vi "SimpleDemo.vi"() -> ()   [LabVIEW 2011]
uses:
  <vilib>/Platform/TimedLoop/XDataNode/timing_clust.ctl
  <vilib>/Platform/TimedLoop/XDataNode/nitl_modes.ctl
  <vilib>/Platform/TimedLoop/XDataNode/wakeup.ctl
  C:/Users/Behavior Room/Desktop/Kinect Mouse/DepthSense/FunctionPointerProxy/FunctionPointerProxy/bin/Release/FunctionPointerProxy.dll
  FunctionPointerProxy/FunctionPointerProxy/bin/Release/FunctionPointerProxy.dll
  <vilib>/Platform/TimedLoop/XDataNode/XDataNode.xnode
  <userlib>/libOptrima-2-3/libOptrima-2-3.lvlib
  <vilib>/Platform/TimedLoop/XDataNode/XDNodeRunTimeDep.lvlib
  Program Files (x86)/SoftKinetic/OptrimaSDK/lib/libOptrima-2-3.dll
panel:
  out "Image 2":T1(plugin-control)
  out "Connect Callback?":i32
  out "Disconnect Callback?":i32
  out "API version":string
  out "NewFrame Callback?":i32
  in  "stop":bool
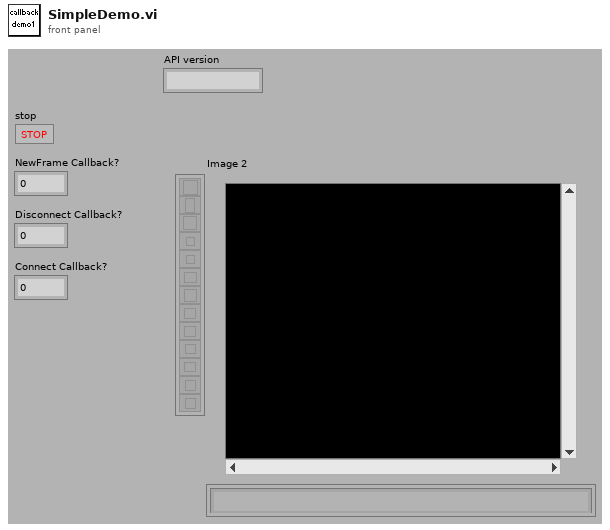
[diagram p1: front panel]
types:
  T1 = typedef "IMAQ Image.ctl" = refnum<image>
  T2 = typedef "t_CallbackReferences.ctl" = cluster{"LV event callback ":refnum<k27>, "Proxy instance":refnum<k24>, "(*f)(...)":i32}
  T3 = cluster{"queue out":refnum<queue>, "queue out":refnum<queue>}
  T4 = typedef "XDNodeRunTimeDep.lvlib/timing_clust.ctl" = cluster{"Expected End [f-1]":u64, "Actual End [f-1]":u64, "Finished Late? [f-1]":bool, "Expected End [i-1]":u64, "Actual End [i-1]":u64, "Finished Late? [i-1]":bool, "Expected Start [i]":u64, "Actual Start [i]":u64, "Expected Start [f]":u64, "Actual Start [f]":u64, "Source Name":string, "Structure Name":string, "Period":i64, "Deadline":i64, "Offset":i64, "Start":i64, "Priority":i32, "Timeout":i32, "Mode":T5, "Wakeup Reason":T6, "Error":errorcluster, "Source Type":string, "Secondary Source Type":string, "Global End Time":u64, "Global Start Time":u64, "Frame Duration":u64, "Iteration Duration":u64, "Assigned CPU":i32, "I/O Scan Engine Mode":u32}
  T5 = typedef "XDNodeRunTimeDep.lvlib/nitl_modes.ctl" = enum32{"No Change", "Process missed periods, maintain original phase", "Discard missed periods, maintain original phase", "Process missed periods, ignore original phase", "Discard missed periods, ignore original phase"}
  T6 = typedef "XDNodeRunTimeDep.lvlib/wakeup.ctl" = enum32{"Normal", "Aborted", "Asynchronous wakeup", "Timing source error", "Timed loop error", "Timeout"}
  T7 = typedef "Image Type" = u32
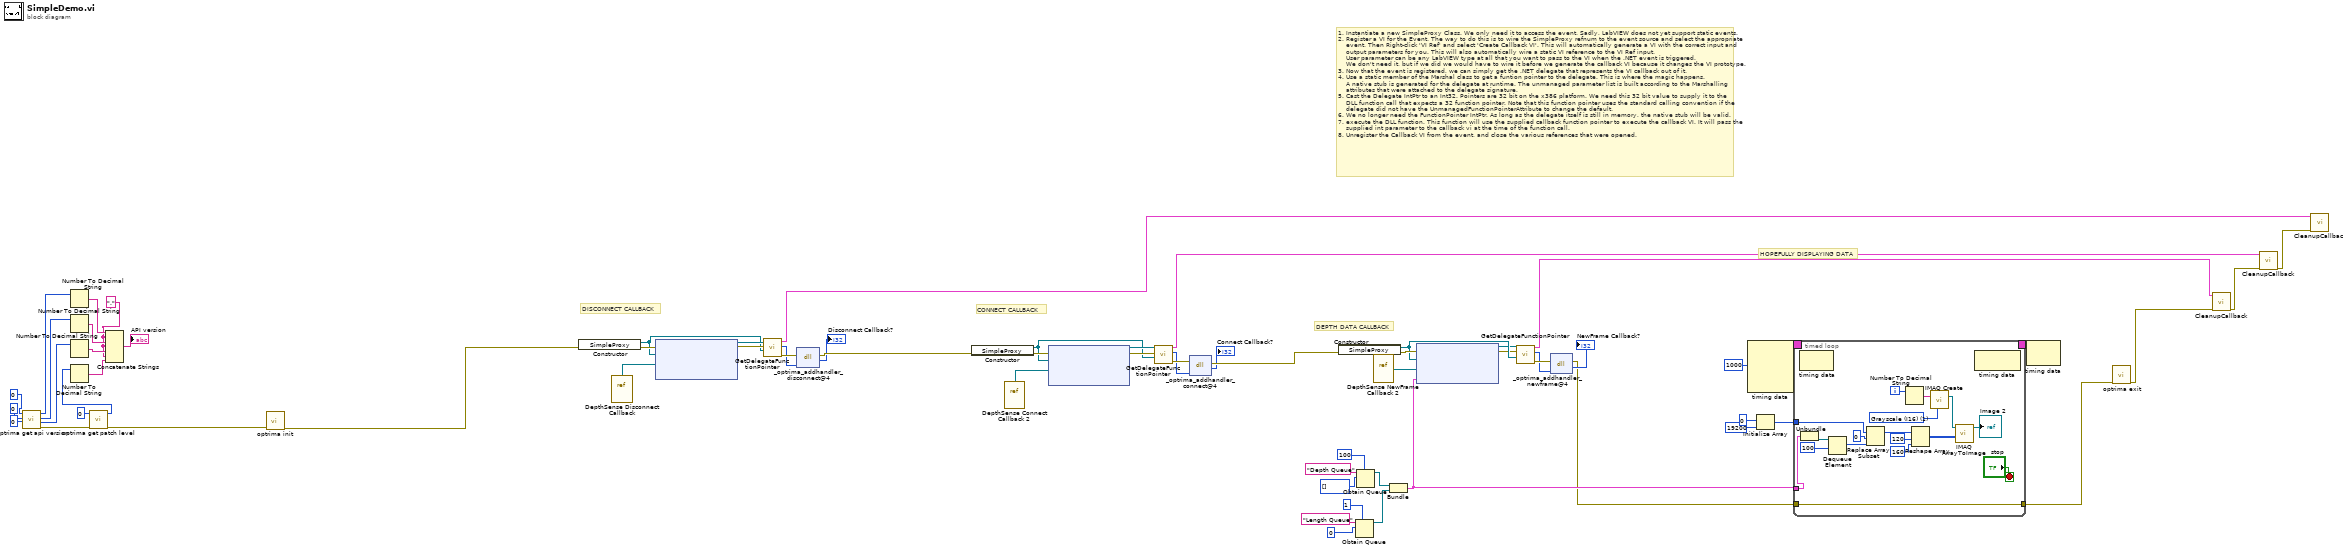
[diagram p0: block diagram]
diagram:
  w44 = "."
  # "HOPEFULLY DISPLAYING DATA"
  # "DEPTH DATA CALLBACK"
  # "CONNECT CALLBACK"
  # "DISCONNECT CALLBACK"
  # "1. Instantiate a new SimpleProxy Class. We only need it to access the event. Sadly, LabVIEW does not yet support static events.\n2. Register a VI for the Event. The way to do this is to wire the SimpleProxy refnum to the event source and select the appropriate\n    event. Then Right-click 'VI Ref' and select 'Create Callback VI'. This will automatically generate a VI with the correct input and\n    output parameters for you. This will also automatically wire a static VI reference to the VI Ref input.\n    User parameter can be any LabVIEW type at all that you want to pass to the VI when the .NET event is triggered.\n    We don't need it, but if we did we would have to wire it before we generate the callback VI because it changes the VI prototype.\n3. Now that the event is registered, we can simply get the .NET delegate that represents the VI callback out of it.\n4. Use a static member of the Marshal class to get a funtion pointer to the delegate. This is where the magic happens.\n    A native stub is generated for the delegate at runtime. The unmanaged parameter list is built according to the Marshalling\n    attributes that were attached to the delegate signature.\n5. Cast the Delegate IntPtr to an Int32. Pointers are 32 bit on the x386 platform. We need this 32 bit value to supply it to the\n    DLL function call that expects a 32 function pointer. Note that this function pointer uses the standard calling convention if the\n    delegate did not have the UnmanagedFunctionPointerAttribute to change the default.\n6. We no longer need the FunctionPointer IntPtr. As long as the delegate itself is still in memory, the native stub will be valid.\n7. execute the DLL function. This function will use the supplied callback function pointer to execute the callback VI. It will pass the\n    supplied int parameter to the callback vi at the time of the function call.\n8. Unregister the Callback VI from the event, and close the various references that were opened."
  n1 = call <userlib>:"optrima get api version.vi"("minor"=u32 0, "major"=u32 0, "release"=u32 0) -> ("error out"=w59:errorcluster, "minor out"=w55:u32, "major out"=w56:u32, "release out"=w57:u32)  [unwired: 5 in]
  n2 = Number To Decimal String(number=w57) -> (decimal integer string=w53:string)  [unwired: 1 in]
  n3 = Number To Decimal String(number=w56) -> (decimal integer string=w47:string)  [unwired: 1 in]
  n4 = Number To Decimal String(number=w55) -> (decimal integer string=w46:string)  [unwired: 1 in]
  n5 = call <userlib>:"optrima get patch level.vi"("error in (no error)"=w59, "patch"=u32 0) -> ("error out"=w58:errorcluster, "patch out"=w54:u32)  [unwired: 8 in]
  n6 = Number To Decimal String(number=w54) -> (decimal integer string=w45:string)  [unwired: 1 in]
  n7 = Concatenate Strings(w53, w44, w47, w44, w46, w44, w45) -> (→"API version":string)
  n8 = call <userlib>:"optrima init.vi"("error in (no error)"=w58) -> ("error out"=w63:errorcluster)  [unwired: 10 in]
  n9 = constructor class="SimpleProxy"(error in=w63) -> (reference out=w37:refnum<k24>, error out=w43:errorcluster)  [unwired: 2 in, 1 out]
  n10 = vi-ref "DepthSense Disconnect Callback.vi"() -> ("vi reference"=w42:refnum<vi>)
  n11 = node(w43, w37, w42) -> (w41:refnum<k27>, w40:errorcluster)  [unwired: 2 in]
  n12 = call "GetDelegateFunctionPointer.vi"("target class"=w37, "error in (no error)"=w40, "event callback refnum"=w41) -> ("error out"=w39:errorcluster, "(*f)(...)"=w38:i32, "References"=w60:T2)  [unwired: 6 in]
  n13 = dll-call lib="C:/Program Files (x86)/SoftKinetic/OptrimaSDK/lib/libOptrima-2-3.dll" fn="_optrima_addhandler_disconnect@4"(error in=w39, "handlerfunc"=w38) -> (error out=w65:errorcluster, "return type"=→"Disconnect Callback?":i32)  [unwired: 3 in, 1 out]
  n14 = constructor class="SimpleProxy"(error in=w65) -> (reference out=w31:refnum<k24>, error out=w35:errorcluster)  [unwired: 2 in, 1 out]
  n15 = vi-ref "DepthSense Connect Callback 2.vi"() -> ("vi reference"=w34:refnum<vi>)
  n16 = node(w35, w31, w34) -> (w33:refnum<k27>, w32:errorcluster)  [unwired: 2 in]
  n17 = call "GetDelegateFunctionPointer.vi"("target class"=w31, "error in (no error)"=w32, "event callback refnum"=w33) -> ("error out"=w30:errorcluster, "(*f)(...)"=w29:i32, "References"=w61:T2)  [unwired: 6 in]
  n18 = dll-call lib="C:/Program Files (x86)/SoftKinetic/OptrimaSDK/lib/libOptrima-2-3.dll" fn="_optrima_addhandler_connect@4"(error in=w30, "handlerfunc"=w29) -> (error out=w64:errorcluster, "return type"=→"Connect Callback?":i32)  [unwired: 3 in, 1 out]
  n19 = constructor class="SimpleProxy"(error in=w64) -> (reference out=w19:refnum<k24>, error out=w27:errorcluster)  [unwired: 2 in, 1 out]
  n20 = Obtain Queue(max queue size (-1, unlimited)=1, name (unnamed)="Length Queue", element data type=0) -> (queue out=w20:refnum<queue>)  [unwired: 2 in, 2 out]
  n21 = Obtain Queue(max queue size (-1, unlimited)=100, name (unnamed)="Depth Queue", element data type=u16[] [] ("p_depthmap in")) -> (queue out=w24:refnum<queue>)  [unwired: 2 in, 2 out]
  n22 = vi-ref "DepthSense NewFrame Callback 2.vi"() -> ("vi reference"=w13:refnum<vi>)
  n23 = Bundle("queue out"=w24, "queue out"=w20) -> (w66:T3)  [unwired: 1 in]
  n24 = node(w27, w19, w13, w66) -> (w17:refnum<k27>, w18:errorcluster)  [unwired: 1 in]
  n25 = call "GetDelegateFunctionPointer.vi"("target class"=w19, "error in (no error)"=w18, "event callback refnum"=w17) -> ("error out"=w16:errorcluster, "(*f)(...)"=w15:i32, "References"=w62:T2)  [unwired: 6 in]
  n26 = dll-call lib="C:/Program Files (x86)/SoftKinetic/OptrimaSDK/lib/libOptrima-2-3.dll" fn="_optrima_addhandler_newframe@4"(error in=w16, "handlerfunc"=w15) -> (error out=w4:errorcluster, "return type"=→"NewFrame Callback?":i32)  [unwired: 3 in, 1 out]
  n27 = node-c288(i64 1000 ("Period")) -> (w11:T4)  [unwired: 3 in]
  n28 = Initialize Array(i16 0 ("element"), 19200 ("dimension size")) -> (w6:i16[])
  n29 = timed-loop {
    tunnel: w66 -> [w82]
    timing: w11 -> [_]
    timing-out: [_] -> w10
    tunnel: w6 -> [w72]
    tunnel: [w67] -> w5
    tunnel: w4 -> [w67]
    i -> [w79]
    stop <- "stop" stop-if-true
    w77 = T7 1 items=["Grayscale (U8)", "Grayscale (I16)", "Grayscale (SGL)", "Complex (CSG)", "RGB (U32)", "HSL (U32)", "RGB (U64)", "Grayscale (U16)"] ("Image Type")
    n30 = node-c288() -> ()  [unwired: 1 in, 1 out]
    n31 = Unbundle(w82) -> ("queue out"=w80:refnum<queue>)  [unwired: 1 out]
    n32 = Dequeue Element(queue=w80, timeout in ms (-1)=100) -> (element=w69:u16[])  [unwired: 1 in, 3 out]
    n33 = Replace Array Subset(array=w72, new element=w69, index=0) -> (w68:i16[])
    n34 = Number To Decimal String(number=w79) -> (decimal integer string=w78:string)  [unwired: 1 in]
    n35 = Reshape Array(w68, 120 ("dimension size"), 160 ("dimension size")) -> (w76:i16[][])
    n36 = call "IMAQ Create"("Image Name"=w78, "Image Type"=w77) -> ("New Image"=w73:T1)  [unwired: 3 in, 1 out]
    n37 = call "IMAQ ArrayToImage"("Image Pixels (I16)"=w76, "Image"=w73) -> ("Image Out"=→"Image 2":T1)  [unwired: 8 in, 1 out]
    n38 = node-c288() -> ()  [unwired: 1 in, 1 out]
  }
  n39 = node-c288(w10) -> ()  [unwired: 1 out]
  n40 = call <userlib>:"optrima exit.vi"("error in (no error)"=w5) -> ("error out"=w3:errorcluster)  [unwired: 10 in]
  n41 = call "CleanupCallback.vi"("error in (no error)"=w3, "References"=w62) -> ("error out"=w2:errorcluster)  [unwired: 9 in]
  n42 = call "CleanupCallback.vi"("error in (no error)"=w2, "References"=w61) -> ("error out"=w1:errorcluster)  [unwired: 9 in]
  n43 = call "CleanupCallback.vi"("error in (no error)"=w1, "References"=w60) -> ()  [unwired: 9 in, 1 out]
